vi "FV_move_rel.vi"(8 "error in":errorcluster, 10 "relative_position":i32, 11 "VISA in":refnum<visa-resource-name>) -> (0 "error out":errorcluster, 3 "VISA out":refnum<visa-resource-name>)   [LabVIEW 2019]
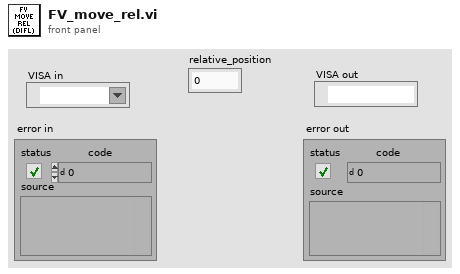
[diagram p1: front panel]
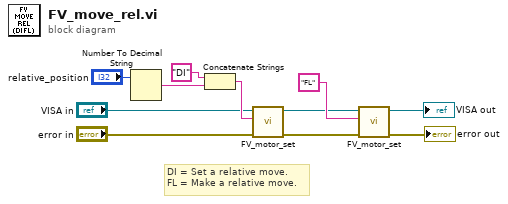
[diagram p0: block diagram]
diagram:
  # "DI = Set a relative move.\nFL = Make a relative move."
  n1 = Number To Decimal String(number="relative_position") -> (decimal integer string=w6:string)  [unwired: 1 in]
  n2 = Concatenate Strings("DI", w6) -> (w11:string)
  n3 = call "FV_motor_set.vi"("error in"="error in", "command"=w11, "VISA in"="VISA in") -> ("error out"=w5:errorcluster, "VISA out"=w1:refnum<visa-resource-name>)  [unwired: 7 in]
  n4 = call "FV_motor_set.vi"("error in"=w5, "command"="FL", "VISA in"=w1) -> ("error out"=→"error out":errorcluster, "VISA out"=→"VISA out":refnum<visa-resource-name>)  [unwired: 7 in]
